vi "Report Cal Measured Power.vi"(0 "CART TCP Connection In":refnum<k5>, 1 "ART2 Version":enum16{"ART2 2.2x", "ART2 4.x"}(ring), 5 "Commit?":bool, 7 "Measured Cal Power":dbl caption="Power", 9 "Chain Mask":u32=1, 11 "error in (no error)":errorcluster, 12 "UL":dbl, 13 "LL":dbl) -> (4 "CART TCP Connection Out":refnum<k5>, 8 "Message Log":string[](array[string]), 10 "Done?":bool, 15 "error out":errorcluster)   [LabVIEW 2012]
uses:
  WLAN Reference/WLAN/UUT/QCA/Controls/QCA NART Message.ctl
  WLAN Reference/WLAN/UUT/QCA/Controls/QCA NART Response Type.ctl
  WLAN Reference/WLAN/UUT/QCA/Controls/QCA NART Response SubType.ctl
  WLAN Reference/WLAN/UUT/QCA/NART Constants.vi
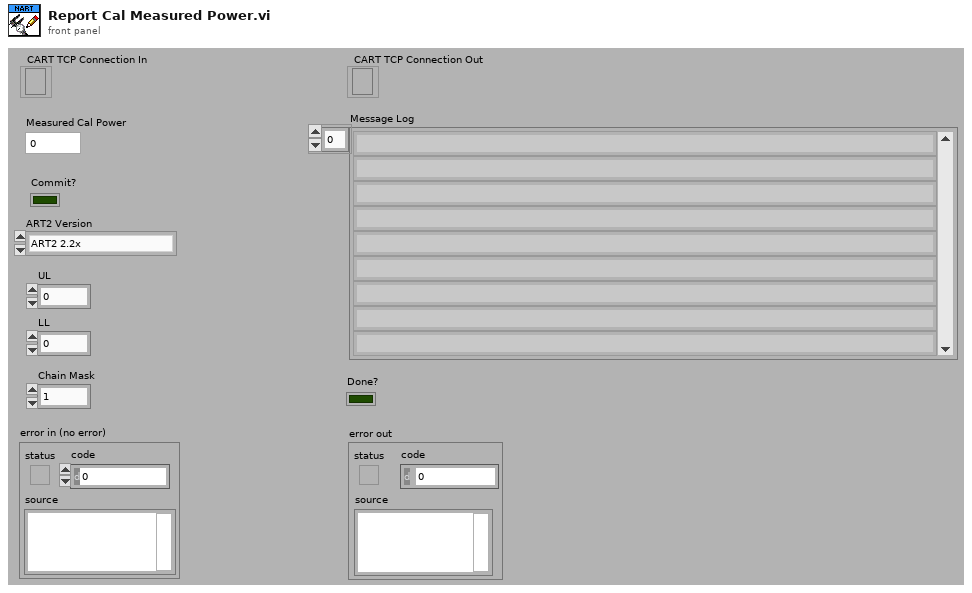
[diagram p1: front panel]
types:
  T1 = cluster{"Name":string, "Type":enum16{"decimal", "string", "float", "hex"}}[]
  T2 = typedef "QCA NART Message.ctl" = cluster{"Code":dbl, "Response Type":T3, "Response Subtype":T4, "Message":string}
  T3 = typedef "QCA NART Response Type.ctl" = enum16{"DEBUG", "CONTROL", "INFO", "WARNING", "ERROR", "NONE"}
  T4 = typedef "QCA NART Response SubType.ctl" = enum16{"NONE", "OK", "ON", "OFF", "BEGIN", "DONE"}
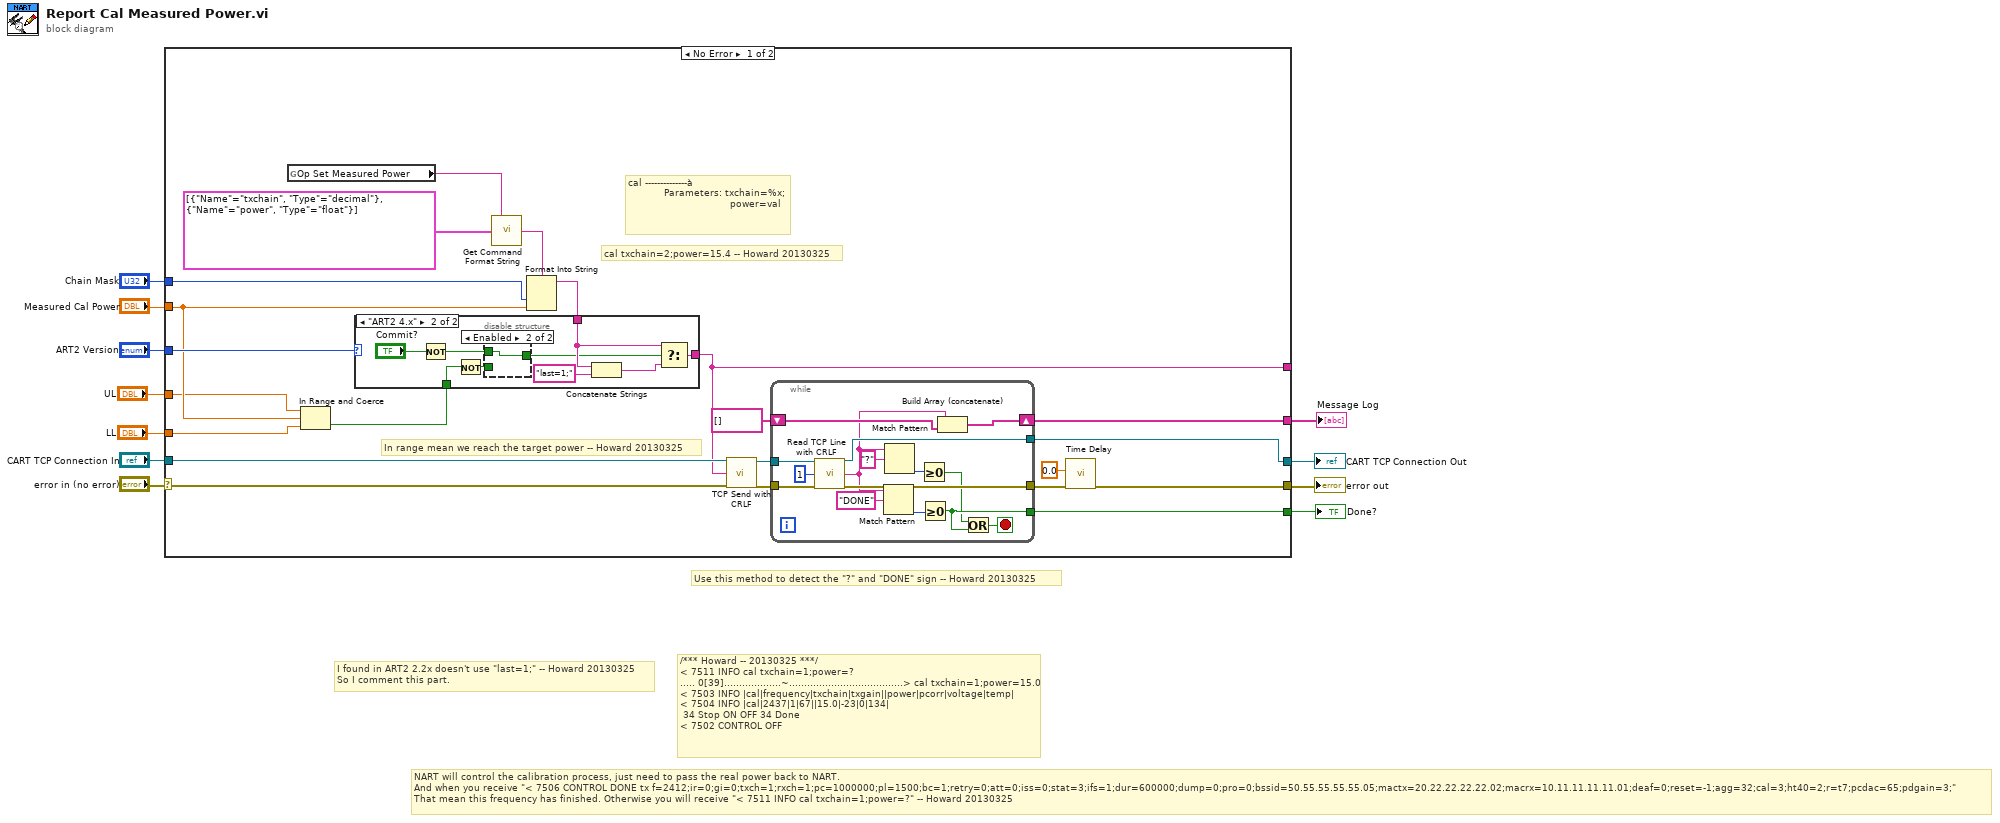
[diagram p0: block diagram]
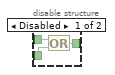
[diagram p3: hidden frame]
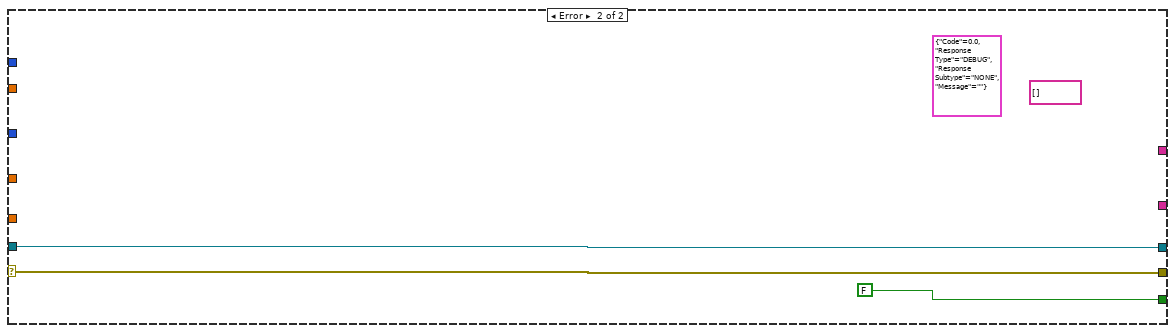
[diagram p4: hidden frame]
diagram:
  # "Use this method to detect the \"?\" and \"DONE\" sign -- Howard 20130325"
  # "NART will control the calibration process, just need to pass the real power back to NART.\nAnd when you receive \"< 7506 CONTROL DONE tx f=2412;ir=0;gi=0;txch=1;rxch=1;pc=1000000;pl=1500;bc=1;retry=0;att=0;iss=0;stat=3;ifs=1;dur=600000;dump=0;pro=0;bssid=50.55.55.55.55.05;mactx=20.22.22.22.22.02;macrx=10.11.11.11.11.01;deaf=0;reset=-1;agg=32;cal=3;ht40=2;r=t7;pcdac=65;pdgain=3;\"\nThat mean this frequency has finished. Otherwise you will receive \"< 7511 INFO cal txchain=1;power=?\" -- Howard 20130325"
  # "/*** Howard -- 20130325 ***/\n< 7511 INFO cal txchain=1;power=?\n..... 0[39]...................~......................................> cal txchain=1;power=15.0\n< 7503 INFO |cal|frequency|txchain|txgain||power|pcorr|voltage|temp|\n< 7504 INFO |cal|2437|1|67||15.0|-23|0|134|\n 34 Stop ON OFF 34 Done\n< 7502 CONTROL OFF"
  # "I found in ART2 2.2x doesn't use \"last=1;\" -- Howard 20130325\nSo I comment this part."
  n1 = case shown="No Error" "error in (no error)" {
    selector: "error in (no error)" -> [w31 w65]
    tunnel: [w14 w65] -> w10
    tunnel: "CART TCP Connection In" -> [w33 w64]
    tunnel: [w13 w64] -> w8
    tunnel: [w18 _] -> w1
    tunnel: "Measured Cal Power" -> [w25 _]
    tunnel: [w28 _] -> _
    tunnel: "ART2 Version" -> [w26 _]
    tunnel: [w20 FALSE] -> w5
    tunnel: "UL" -> [w24 _]
    tunnel: "LL" -> [w23 _]
    tunnel: "Chain Mask" -> [w17 _]
    frame No Error {
      # "In range mean we reach the target power -- Howard 20130325"
      # "cal txchain=2;power=15.4 -- Howard 20130325"
      # "cal --------------à\n            Parameters: txchain=%x;\n                                  power=val"
      n2 = global read "NART Constants.vi" "Op Set Measured Power"() -> (w30:string)
      n3 = In Range and Coerce(upper limit=w24, x=w25, lower limit=w23) -> (In Range?=w16:bool)  [unwired: 1 out]
      n4 = call "Get Command Format String.vi"("Command"=w30, "Parameters"=T1 [{"Name"="txchain", "Type"=enum."decimal"}, {"Name"="power", "Type"=enum."float"}]) -> ("Command Format String"=w29:string)  [unwired: 13 in]
      n5 = Format Into String(format string=w29, w17, w25) -> (resulting string=w27:string)  [unwired: 2 in, 1 out]
      n6 = case shown="\"ART2 4.x\"" w26 {
        tunnel: [w49 w58] -> w28
        tunnel: w27 -> [w49 w55]
        tunnel: w16 -> [_ w52]
        frame "ART2 2.2x", Default {
        }
        frame "ART2 4.x" {
          n7 = Not(x="Commit?") -> (.not. x?=w53:bool)
          n8 = Not(x=w52) -> (.not. x?=w50:bool)
          n9 = disable-structure shown="Enabled" {
            disable-tunnel: w53 -> [w61 w62]
            disable-tunnel: [w60 w62] -> w51
            disable-tunnel: w50 -> [w59 _]
            frame Disabled {
              n10 = Or(x=w61, y=w59) -> (x .or. y?=w60:bool)
            }
            frame Enabled {
            }
          }
          n11 = Concatenate Strings(w55, "last=1;" ("string")) -> (w54:string)
          n12 = Select(t=w55, s=w51, f=w54) -> (s? t:f=w58:string)
        }
      }
      n13 = call "TCP Send with CRLF.vi"("CART TCP Connection"=w33, "data in"=w28, "error IO"=w31) -> ("CART TCP Connection Out"=w21:refnum<k5>, "error out"=w22:errorcluster)  [unwired: 11 in]
      n14 = while {
        tunnel: w22 -> [w48]
        tunnel: w21 -> [w47]
        tunnel: [w41] -> w20
        tunnel: [w40] -> w19
        tunnel: [w38] -> w13
        shift-right: [w37] -> w18
        shift-left: string[] [] -> [w35]
        stop <- w39 stop-if-true
        n15 = call "Read TCP Line with CRLF.vi"("TCP Connection In"=w47, "timeout ms (100)"=1, "error in"=w48) -> ("TCP Connection Out"=w38:refnum<k5>, "TCP Line"=w34:string, "error out"=w40:errorcluster)  [unwired: 10 in]
        n16 = Match Pattern(string=w34, regular expression="DONE") -> (offset past match=w42:i32)  [unwired: 1 in, 3 out]
        n17 = Match Pattern(string=w34, regular expression="?") -> (offset past match=w43:i32)  [unwired: 1 in, 3 out]
        n18 = Greater Or Equal To 0?(x=w43) -> (x >= 0?=w36:bool)
        n19 = Greater Or Equal To 0?(x=w42) -> (x >= 0?=w41:bool)
        n20 = Build Array (concatenate)(w34, w35) -> (w37:string[])
        n21 = Or(x=w36, y=w41) -> (x .or. y?=w39:bool)
      }
      n22 = call "Time Delay"("error in (no error)"=w19, "Delay Time (s)"=0.0) -> ("error out"=w14:errorcluster)  [unwired: 9 in]
    }
    frame Error {
      (unwired) T2 {"Code"=0.0, "Response Type"=enum."DEBUG", "Response Subtype"=enum."NONE", "Message"=""} ("Desired Response")
      (unwired) string[] [] ("TCP Messages")
    }
  }
  "error out" <- w10
  "CART TCP Connection Out" <- w8
  "Done?" <- w5
  "Message Log" <- w1
